vi "sv_Order Mag and Phase with DFT (N Freq, 1 Ch).vi"(0 "buffered x[n]":dbl[](array[numeric]) format="%.2f", 5 "fs":i32=1, 9 "fc [Hz]":dbl[](array[numeric])=[0.0] format="%.2f") -> (4 "mag [RMS]":dbl[](array[numeric]), 6 "phase":dbl[](array[numeric]))   [LabVIEW 2017]
uses:
  <vilib>/Analysis/4window.llb/windowTd.ctl
  <vilib>/Analysis/baseanly.llb/Mean (DBL).vi
  <vilib>/Analysis/0measdsp.llb/Scaled Time Domain Window (DBL).vi
  <vilib>/addons/Sound and Vibration/Order Analysis/Resample Order Tracking/SoundVib_Resampling.lvlib
  <vilib>/Analysis/NI_AALPro.lvlib
  <vilib>/Analysis/NI_AALBase.lvlib
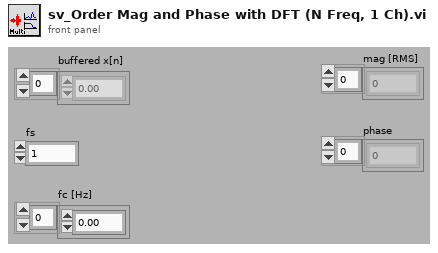
[diagram p1: front panel]
types:
  T1 = typedef "NI_AALPro.lvlib/windowTd.ctl" = u32
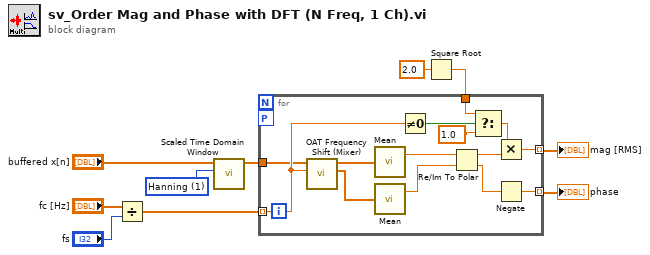
[diagram p0: block diagram]
diagram:
  w3 = T1 1 items=["Rectangle"=0, "Hanning"=1, "Hamming"=2, "Blackman-Harris"=3, "Exact Blackman"=4, "Blackman"=5, "Flat Top"=6, "4 Term B-Harris "=7, "7 Term B-Harris"=8, "Low Sidelobe"=9, "Blackman Nuttall"=11, "Triangle"=30, "Bartlett-Hanning"=31, "Bohman"=32, "Parzen"=33, "Welch"=34, "Kaiser"=60, "Dolph-Chebyshev"=61, "Gaussian"=62] ("window")
  n1 = Divide(x="fc [Hz]", y="fs") -> (x/y=w10:dbl[])
  n2 = call-poly <vilib>:"Scaled Time Domain Window.vi"("window"=w3, "X"="buffered x[n]") -> ("Windowed X"=w2:dbl[])  [unwired: 7 in, 2 out]
  n3 = Square Root(x=2.0) -> (sqrt(x)=w8:dbl)
  n4 = for {
    tunnel: w10 -> [w22] mode=indexing
    tunnel: w8 -> [w20]
    tunnel: [w16] -> w4 mode=indexing
    tunnel: [w17] -> w5 mode=indexing
    tunnel: w2 -> [w11]
    workers-P: _ -> [_]
    n5 = call <vilib>:"OAT Frequency Shift (Mixer).vi"("fc"=w22, "X"=w11) -> ("imaginary"=w15:dbl[], "real"=w12:dbl[])  [unwired: 7 in, 1 out]
    n6 = call-poly <vilib>:"Mean.vi"("X"=w12) -> ("mean"=w14:dbl)  [unwired: 1 out]
    n7 = call-poly <vilib>:"Mean.vi"("X"=w15) -> ("mean"=w13:dbl)  [unwired: 1 out]
    n8 = Not Equal To 0?(x=w22) -> (x != 0?=w21:bool)
    n9 = Re/Im To Polar(2:w13, 3:w14) -> (0:w23:dbl, 1:w24:dbl)
    n10 = Select(t=w20, s=w21, f=1.0) -> (s? t:f=w19:dbl)
    n11 = Multiply(x=w19, y=w24) -> (x*y=w17:dbl)
    n12 = Negate(x=w23) -> (-x=w16:dbl)
  }
  "mag [RMS]" <- w5
  "phase" <- w4
